vi "Initialize.vi"(8 "error in (no error)":errorcluster, 10 "Circular Buffer Size":i32=10, 11 "Data Plugin in":refnum<class "Data Plugin.lvclass">) -> (0 "error out":errorcluster, 3 "Data Plugin out":refnum<class "Data Plugin.lvclass">)   [LabVIEW 2017, in "Data Engine.lvlib" / "Data Plugin.lvclass"]
uses:
  Data Plugin.lvclass
  Data Plugin.lvclass/Data Plugin.ctl
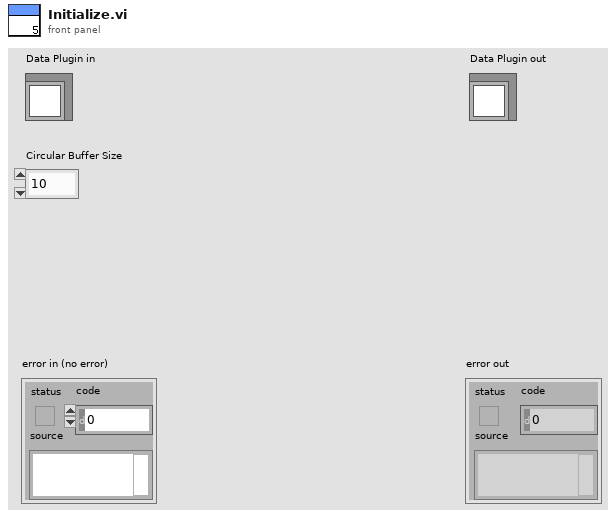
[diagram p1: front panel]
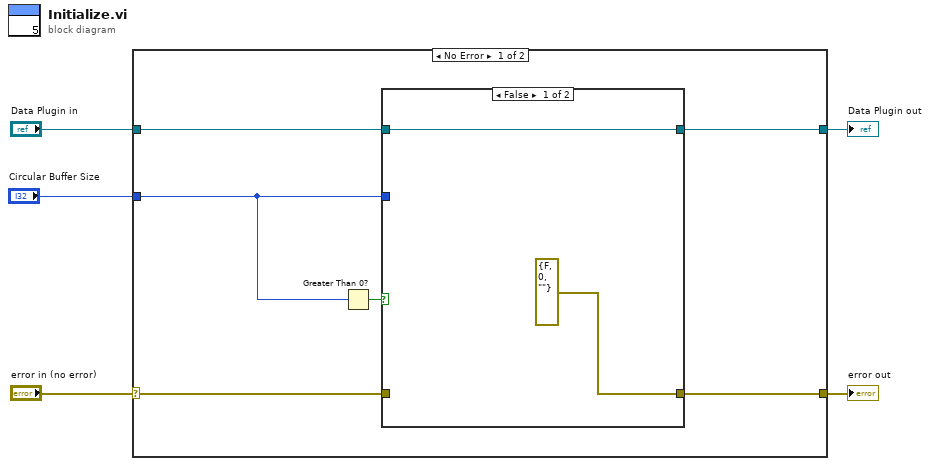
[diagram p0: block diagram]
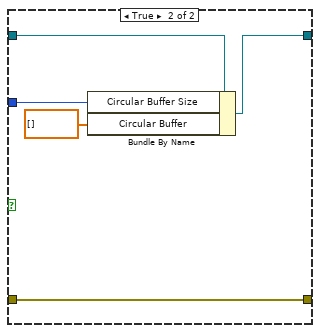
[diagram p2: hidden frame]
diagram:
  n1 = case shown="No Error" "error in (no error)" {
    selector: "error in (no error)" -> [w6 w20]
    tunnel: [w7 w20] -> w4
    tunnel: [w10 w19] -> w2
    tunnel: "Data Plugin in" -> [w11 w19]
    tunnel: "Circular Buffer Size" -> [w9 _]
    frame No Error {
      n2 = Greater Than 0?(x=w9) -> (x > 0?=w8:bool)
      n3 = case shown="False" w8 {
        tunnel: w11 -> [w13 w18]
        tunnel: [w13 w14] -> w10
        tunnel: w9 -> [_ w16]
        tunnel: [errorcluster {"status"=FALSE, "code"=0, "source"=""} ("error IO") w15] -> w7
        tunnel: w6 -> [_ w15]
        frame False {
        }
        frame True {
          n4 = Bundle By Name(cluster=w18, "Circular Buffer Size"=w16, "Circular Buffer"=dbl[] []) -> (w14:refnum<class "Data Plugin.lvclass">)
        }
      }
    }
    frame Error {
    }
  }
  "error out" <- w4
  "Data Plugin out" <- w2
